vi "Init UI.vi"(8 "error in (no error)":errorcluster, 11 "Mixer in":refnum<class "Transport.lvclass">) -> (0 "error out":errorcluster, 3 "Mixer out":refnum<class "Transport.lvclass">)   [LabVIEW 2020, in "Transport.lvclass"]
uses:
  Transport.lvclass
  Transport.lvclass/Transport.ctl
  Packed Libraries/Messaging.lvlibp
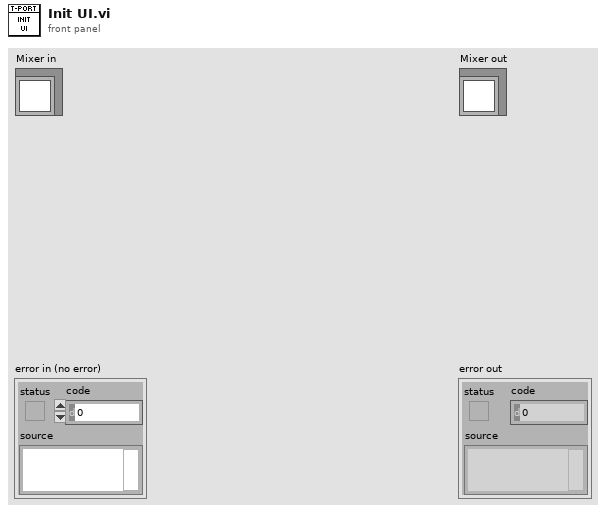
[diagram p1: front panel]
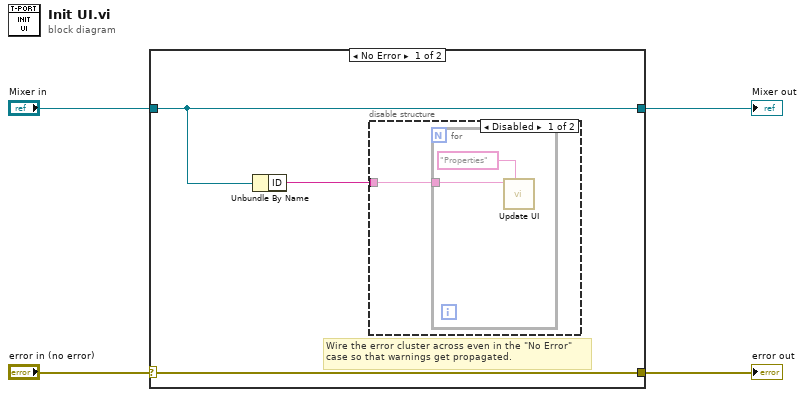
[diagram p0: block diagram]
diagram:
  n1 = case shown="No Error" "error in (no error)" {
    selector: "error in (no error)" -> [w7 w12]
    tunnel: [w7 w12] -> w2
    tunnel: [w6 w11] -> w1
    tunnel: "Mixer in" -> [w6 w11]
    frame No Error {
      # "Wire the error cluster across even in the \"No Error\"\ncase so that warnings get propagated."
      n2 = Unbundle By Name(w6) -> ("ID"=w5:string)
      n3 = disable-structure shown="Disabled" {
        disable-tunnel: w5 -> [w8 _]
        frame Disabled {
          n4 = for {
            tunnel: w8 -> [w10]
            n5 = call "Update UI.vi"("Message (Value Change)"="Properties", "ID"=w10) -> ()  [unwired: 9 in, 1 out]
          }
        }
        frame Enabled {
        }
      }
    }
    frame Error {
    }
  }
  "error out" <- w2
  "Mixer out" <- w1
